vi "Output OFF.vi"(8 "error in (no error)":errorcluster, 11 "VISA resource name":refnum<visa-resource-name>) -> (0 "value out":errorcluster, 3 "VISA resource name out":refnum<visa-resource-name>)   [LabVIEW 2023, in "TDK20-38 API.lvlib"]
uses:
  TDK20-38 API.lvlib
  d553cda4-a0a5-4922-8397-6d23ad06ce71.vi
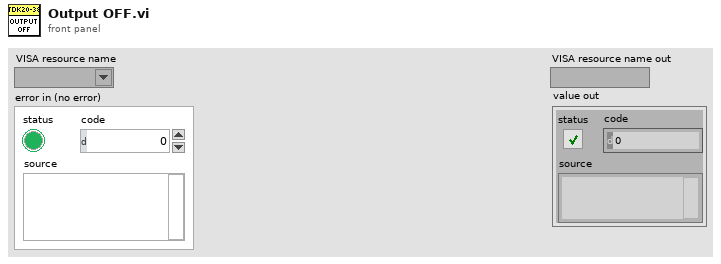
[diagram p1: front panel]
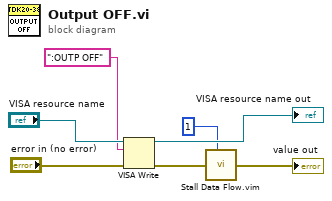
[diagram p0: block diagram]
diagram:
  n1 = VISA Write(VISA resource name="VISA resource name", write buffer=":OUTP OFF" ("format string"), error in (no error)="error in (no error)") -> (VISA resource name out=→"VISA resource name out":refnum<visa-resource-name>, error out=w4:errorcluster)  [unwired: 1 out]
  n2 = call "Stall Data Flow.vim"("value in"=w4, "milliseconds to wait"=u32 1) -> ("value out"=→"value out":errorcluster)  [unwired: 1 out]
